vi "AutoArray.vi"(0 "Array":dbl[][](array[numeric])) -> ()   [LabVIEW 2017]
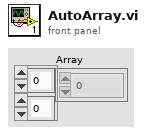
[diagram p1: front panel]
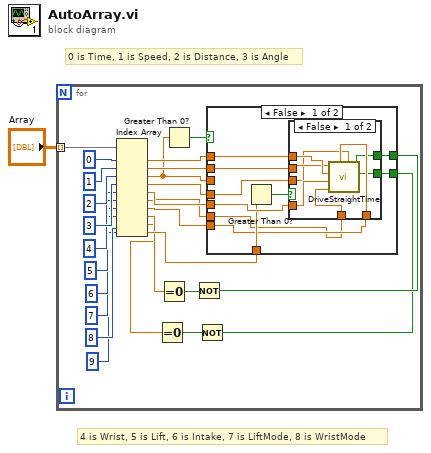
[diagram p0: block diagram]
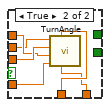
[diagram p2: hidden frame]
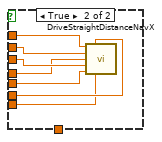
[diagram p3: hidden frame]
diagram:
  # "4 is Wrist, 5 is Lift, 6 is Intake, 7 is LiftMode, 8 is WristMode"
  # "0 is Time, 1 is Speed, 2 is Distance, 3 is Angle"
  n1 = for {
    tunnel: "Array" -> [w27] mode=indexing
    n2 = Index Array(array=w27, index #1=0 ("index"), index #2=1 ("index"), index #3=2 ("index"), index #4=3 ("index"), index #5=4 ("index"), index #6=5 ("index"), index #7=6 ("index"), index #8=7 ("index"), index #9=8 ("index"), index #10=9 ("index")) -> (element #1=w20:dbl, element #2=w21:dbl, element #3=w18:dbl, element #4=w19:dbl, element #5=w13:dbl, element #6=w12:dbl, element #7=w11:dbl, element #8=w4:dbl, element #9=w3:dbl, element #10=w9:dbl)
    n3 = Equal To 0?(x=w3) -> (x = 0?=w7:bool)
    n4 = Equal To 0?(x=w4) -> (x = 0?=w8:bool)
    n5 = Greater Than 0?(x=w18) -> (x > 0?=w22:bool)
    n6 = Not(x=w8) -> (.not. x?=w6:bool)
    n7 = Not(x=w7) -> (.not. x?=w5:bool)
    n8 = case shown="False" w22 {
      tunnel: w21 -> [w35 w58]
      tunnel: w20 -> [w36 w52]
      tunnel: w18 -> [_ w57]
      tunnel: w19 -> [w34 w56]
      tunnel: w13 -> [w33 w55]
      tunnel: w12 -> [w30 w54]
      tunnel: w11 -> [w31 w53]
      tunnel: w9 -> [w32 _]
      tunnel: w6 -> [w29 _]
      tunnel: w5 -> [w28 _]
      frame False {
        n9 = Greater Than 0?(x=w32) -> (x > 0?=w37:bool)
        n10 = case shown="False" w37 {
          tunnel: w36 -> [w42 w50]
          tunnel: w35 -> [w41 w48]
          tunnel: w34 -> [w40 w51]
          tunnel: w33 -> [w45 w49]
          tunnel: w31 -> [w43 w46]
          tunnel: w30 -> [w44 w47]
          tunnel: w29 -> [w39 _]
          tunnel: w28 -> [w38 _]
          frame False {
            n11 = call "DriveStraightTime.vi"("WristMode"=w38, "LiftMode"=w39, "Angle"=w40, "Intake"=w43, "Lift"=w44, "Wrist"=w45, "Time"=w42, "Speed"=w41) -> ()  [unwired: 3 in]
          }
          frame True {
            n12 = call "TurnAngle.vi"("Intake"=w46, "Lift"=w47, "Wrist"=w49, "Time"=w50, "AngleSetpoint"=w51, "MaxSpeed"=w48) -> ()  [unwired: 5 in]
          }
        }
      }
      frame True {
        n13 = call "DriveStraightDistanceNavX.vi"("Time"=w52, "Lift"=w54, "Speed"=w58, "Angle"=w56, "Distance"=w57, "Wrist"=w55, "Intake"=w53) -> ()  [unwired: 9 in]
      }
    }
  }
